vi "Convert with Linear Calibration (1D, DBL).vi"(10 "Linear Calibration 1D":T1, 11 "A":dbl) -> (3 "A*":dbl)   [LabVIEW 2011, in "COSYLib.lvlib"]
doc: "Calculates Y=AX+B, with A and B taken from a <B>Linear Calibration</B> cluster."
uses:
  Linear Calibration 1D.ctl
  COSYLib.lvlib
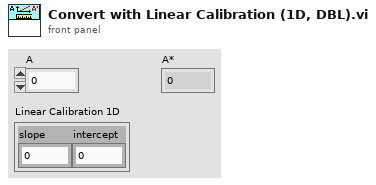
[diagram p1: front panel]
types:
  T1 = typedef "COSYLib.lvlib/Linear Calibration 1D.ctl" = cluster{"slope":dbl, "intercept":dbl}
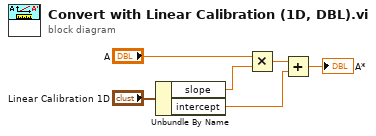
[diagram p0: block diagram]
diagram:
  n1 = Unbundle By Name("Linear Calibration 1D") -> ("slope"=w4:dbl, "intercept"=w2:dbl)
  n2 = Multiply(x="A", y=w4) -> (x*y=w3:dbl)
  n3 = Add(x=w3, y=w2) -> (x+y=→"A*":dbl)
